vi "Handle.vi"(8 "error in (no error)":errorcluster, 11 "GSserver in":refnum<class "GSserver.lvclass">) -> (0 "error out":errorcluster, 3 "GSserver out":refnum<class "GSserver.lvclass">)   [LabVIEW 2018, in "GSserver.lvclass"]
uses:
  GSserver.lvclass
  C:/Users/observer/Desktop/Sparc4GUI/Versao ZeroMQ/SPARC4_GUI - projeto para EXE - Desenv/Server/Server.lvclass
  GSserver.lvclass/GSserver.ctl
  Device/Device.lvclass/Device.ctl
  Server/Server.lvclass/Server.ctl
  GSstatus/GSstatus.lvclass
  C:/Users/observer/Desktop/Sparc4GUI/Versao ZeroMQ/SPARC4_GUI - projeto para EXE - Desenv/Device/Device.lvclass
  Server/Server.lvclass
  Comm/Stream/Stream.lvclass
  Device/Device.lvclass
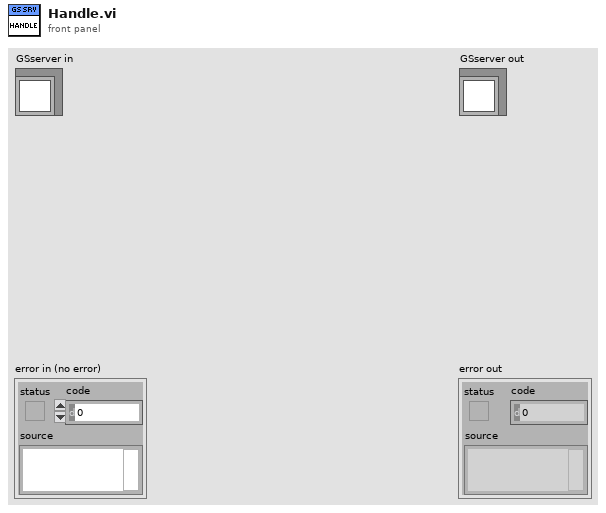
[diagram p1: front panel]
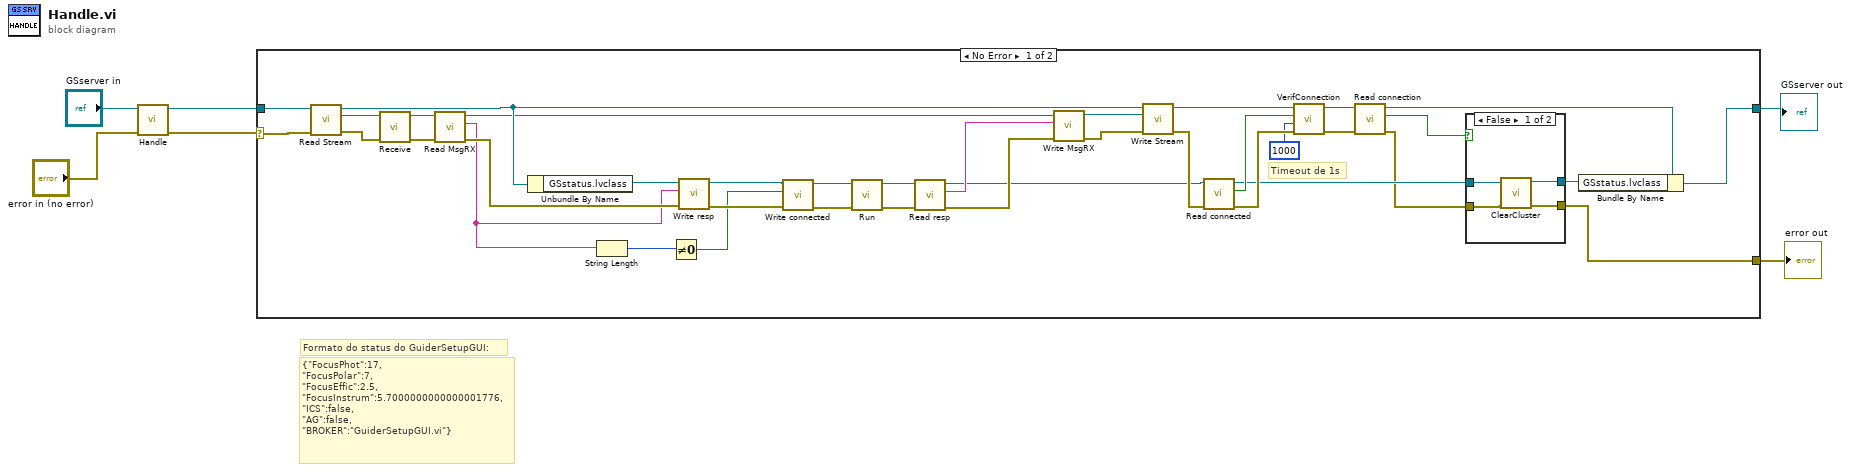
[diagram p0: block diagram]
diagram:
  # "Formato do status do GuiderSetupGUI:"
  # "{\"FocusPhot\":17,\n\"FocusPolar\":7,\n\"FocusEffic\":2.5,\n\"FocusInstrum\":5.7000000000000001776,\n\"ICS\":false,\n\"AG\":false,\n\"BROKER\":\"GuiderSetupGUI.vi\"}"
  n1 = call-parent "Handle.vi"("error in (no error)"="error in (no error)", "Server in"="GSserver in") -> ("error out"=w3:errorcluster, "Server out"=w4:refnum<class "GSserver.lvclass">)  [unwired: 8 in]
  n2 = case shown="No Error" w3 {
    selector: w3 -> [w42 w52]
    tunnel: [w7 w52] -> w2
    tunnel: [w41 w51] -> w1
    tunnel: w4 -> [w37 w51]
    frame No Error {
      # "Timeout de 1s"
      n3 = call-dynamic "Read Stream.vi"("error in (no error)"=w42, "Server in"=w37) -> ("error out"=w43:errorcluster, "Stream.lvclass"=w44:refnum<class "Stream.lvclass">, "Server out"=w29:refnum<class "GSserver.lvclass">)  [unwired: 7 in]
      n4 = call-dynamic "Receive.vi"("error in (no error)"=w43, "Stream in"=w44) -> ("error out"=w40:errorcluster, "Stream out"=w39:refnum<class "Stream.lvclass">)  [unwired: 8 in]
      n5 = call-dynamic "Read MsgRX.vi"("error in (no error)"=w40, "Comm in"=w39) -> ("error out"=w38:errorcluster, "MsgRX"=w35:string, "Comm out"=w18:refnum<class "Stream.lvclass">)  [unwired: 7 in]
      n6 = Unbundle By Name(w29) -> ("GSstatus.lvclass"=w28:refnum<class "GSstatus.lvclass">)
      n7 = String Length(string=w35) -> (length=w36:i32)
      n8 = Not Equal To 0?(x=w36) -> (x != 0?=w23:bool)
      n9 = call-dynamic "Write resp.vi"("error in (no error)"=w38, "resp"=w35, "Device in"=w28) -> ("error out"=w25:errorcluster, "Device out"=w27:refnum<class "GSstatus.lvclass">)  [unwired: 7 in]
      n10 = call "Write connected.vi"("error in (no error)"=w25, "connected"=w23, "Device in"=w27) -> ("error out"=w24:errorcluster, "Device out"=w26:refnum<class "GSstatus.lvclass">)  [unwired: 7 in]
      n11 = call-dynamic "Run.vi"("error in (no error)"=w24, "GSstatus in"=w26) -> ("error out"=w22:errorcluster, "GSstatus out"=w21:refnum<class "GSstatus.lvclass">)  [unwired: 8 in]
      n12 = call-dynamic "Read resp.vi"("error in (no error)"=w22, "Device in"=w21) -> ("error out"=w20:errorcluster, "resp"=w19:string, "Device out"=w15:refnum<class "GSstatus.lvclass">)  [unwired: 7 in]
      n13 = call-dynamic "Write MsgRX.vi"("error in (no error)"=w20, "MsgRX"=w19, "Comm in"=w18) -> ("error out"=w16:errorcluster, "Comm out"=w17:refnum<class "Stream.lvclass">)  [unwired: 7 in]
      n14 = call-dynamic "Write Stream.vi"("error in (no error)"=w16, "Stream.lvclass"=w17, "Server in"=w29) -> ("error out"=w34:errorcluster, "Server out"=w33:refnum<class "GSserver.lvclass">)  [unwired: 7 in]
      n15 = call "Read connected.vi"("error in (no error)"=w34, "Device in"=w15) -> ("error out"=w31:errorcluster, "connected"=w32:bool, "Device out"=w10:refnum<class "GSstatus.lvclass">)  [unwired: 7 in]
      n16 = call-dynamic "VerifConnection.vi"("error in (no error)"=w31, "timeout in ms (1000)"=u32 1000 ("period (ms)"), "device connected in"=w32, "Server in"=w33) -> ("error out"=w12:errorcluster, "Server out"=w13:refnum<class "GSserver.lvclass">)  [unwired: 6 in]
      n17 = call "Read connection.vi"("error in (no error)"=w12, "Server in"=w13) -> ("error out"=w8:errorcluster, "connection"=w14:bool, "Server out"=w11:refnum<class "GSserver.lvclass">)  [unwired: 7 in]
      n18 = case shown="False" w14 {
        tunnel: [w47 w50] -> w9
        tunnel: w10 -> [w48 w50]
        tunnel: w8 -> [w46 w49]
        tunnel: [w45 w49] -> w7
        frame False {
          n19 = call-dynamic "ClearCluster.vi"("error in (no error)"=w46, "GSstatus in"=w48) -> ("error out"=w45:errorcluster, "GSstatus out"=w47:refnum<class "GSstatus.lvclass">)  [unwired: 8 in]
        }
        frame True {
        }
      }
      n20 = Bundle By Name(cluster=w11, "GSstatus.lvclass"=w9) -> (w41:refnum<class "GSserver.lvclass">)
    }
    frame Error {
    }
  }
  "error out" <- w2
  "GSserver out" <- w1
